vi "Periodic Tasks.vi"(8 "error in":errorcluster) -> ()   [LabVIEW 2018]
doc: "This VI runs in parallel to other robot code. It can contain as many user-defined periodic loops as you need. These can carry out PID or other sorts of timed response."
uses:
  <vilib>/Rock Robotics/WPI/Utilities/WPI_GetSetVariantRefNum.vi
  Robot Global Data.vi
panel:
  out "Cargo Stop Current":dbl=10.0 format="%#_13g"
  out "Stop the grabber":bool
  out "Solenoid Voltage":dbl
  out "Input Voltage":dbl
  out "Compressor current (A)":dbl
  out "all currents (A)":dbl[](array[numeric]) caption="0\n1\n2\n3\n4\n5\n6\n7\n8\n9\n10\n11\n12\n13\n14\n15"
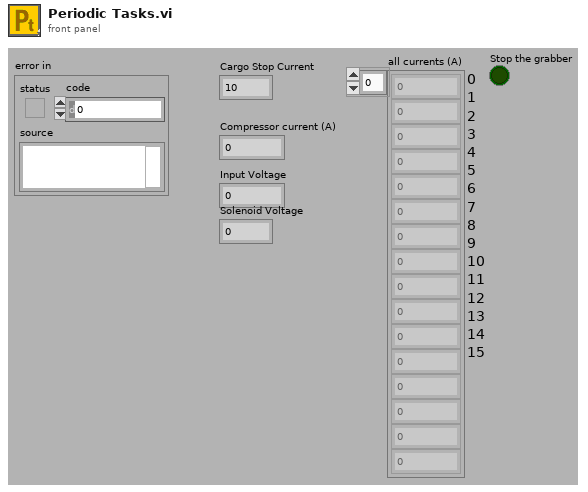
[diagram p1: front panel]
types:
  T1 = typedef "WPI_JoystickDevRef.ctl" = cluster{"Device":T2}
  T2 = typedef "WPI_JoystickDeviceEnum.ctl" = enum16{"USB 0", "USB 1", "USB 2", "USB 3", "USB 4", "USB 5"}
  T3 = cluster{"JoystickDevRef":T1, "JoystickDevRef":T1}
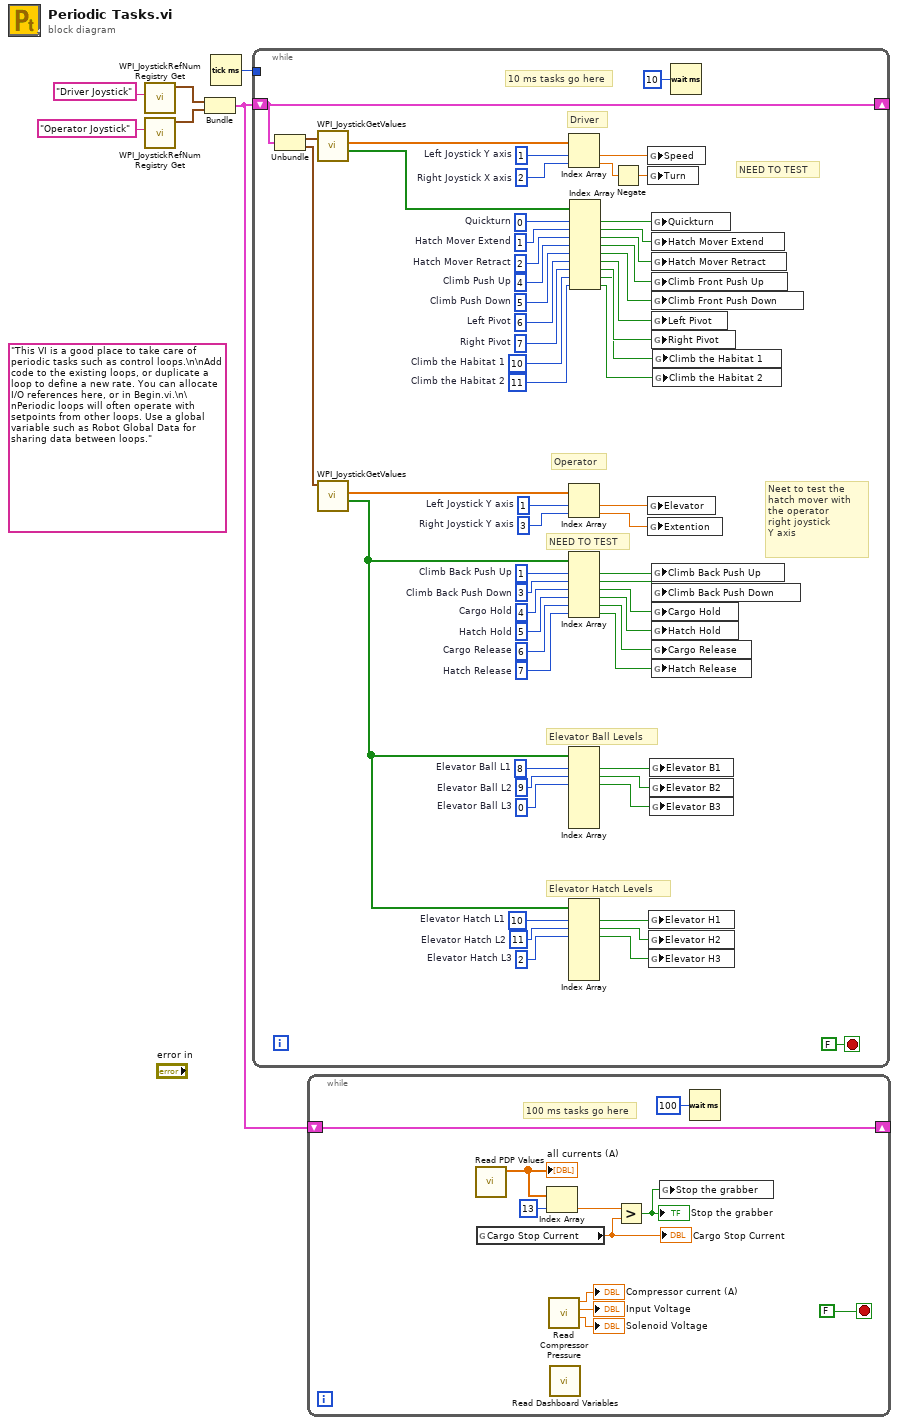
[diagram p0: block diagram]
diagram:
  (unwired) "This VI is a good place to take care of periodic tasks such as control loops.\n\nAdd code to the existing loops, or duplicate a loop to define a new rate. You can allocate I/O references here, or in Begin.vi.\n\nPeriodic loops will often operate with setpoints from other loops. Use a global variable such as Robot Global Data for sharing data between loops."
  n1 = call <vilib>:"WPI_JoystickRefNum Registry Get.vi"("refnum name"="Driver Joystick") -> ("JoystickDevRef"=w3:T1)  [unwired: 1 in, 9 out]
  n2 = call <vilib>:"WPI_JoystickRefNum Registry Get.vi"("refnum name"="Operator Joystick") -> ("JoystickDevRef"=w1:T1)  [unwired: 1 in, 9 out]
  n3 = Bundle("JoystickDevRef"=w3, "JoystickDevRef"=w1) -> (w2:T3)  [unwired: 1 in]
  n4 = Tick Count (ms)() -> (millisecond timer value=w5:u32)
  n5 = while {
    shift-right: [w61] -> _
    shift-left: w2 -> [w61]
    tunnel: w5 -> [_]
    stop <- FALSE stop-if-true
    w7 = 11  # Climb the Habitat 2
    w10 = 10  # Climb the Habitat 1
    w15 = 2  # Elevator Hatch L3
    w16 = 11  # Elevator Hatch L2
    w17 = 10  # Elevator Hatch L1
    w20 = 0  # Elevator Ball L3
    w19 = 9  # Elevator Ball L2
    w18 = 8  # Elevator Ball L1
    w25 = 3  # Right Joystick Y axis
    w29 = 7  # Right Pivot
    w28 = 6  # Left Pivot
    w35 = 5  # Climb Push Down
    w36 = 4  # Climb Push Up
    w43 = 7  # Hatch Release
    w44 = 6  # Cargo Release
    w45 = 5  # Hatch Hold
    w46 = 4  # Cargo Hold
    w47 = 3  # Climb Back Push Down
    w48 = 1  # Climb Back Push Up
    w50 = 1  # Left Joystick Y axis
    w51 = 2  # Hatch Mover Retract
    w52 = 1  # Hatch Mover Extend
    w53 = 0  # Quickturn
    w56 = 2  # Right Joystick X axis
    w57 = 1  # Left Joystick Y axis
    # "Elevator Hatch Levels"
    # "Elevator Ball Levels"
    # "10 ms tasks go here"
    # "Neet to test the\nhatch mover with\nthe operator \nright joystick\nY axis"
    # "Operator"
    # "Driver"
    # "NEED TO TEST"
    # "NEED TO TEST"
    n6 = Unbundle(w61) -> ("JoystickDevRef"=w60:T1, "JoystickDevRef"=w58:T1)
    n7 = call <vilib>:"WPI_JoystickGetValues.vi"("JoystickDevRef"=w60) -> ("Buttons"=w62:bool[], "Axes"=w64:dbl[])  [unwired: 6 in, 3 out]
    n8 = call <vilib>:"WPI_JoystickGetValues.vi"("JoystickDevRef"=w58) -> ("Buttons"=w11:bool[], "Axes"=w59:dbl[])  [unwired: 6 in, 3 out]
    n9 = Index Array(array=w64, index #1=w57, index #2=w56) -> (element #1=w55:dbl, element #2=w54:dbl)
    n10 = Index Array(array=w59, index #1=w50, index #2=w25) -> (element #1=w49:dbl, element #2=w24:dbl)
    n11 = Index Array(array=w11, index #1=w48, index #2=w47, index #3=w46, index #4=w45, index #5=w44, index #6=w43) -> (element #1=w42:bool, element #2=w41:bool, element #3=w40:bool, element #4=w39:bool, element #5=w38:bool, element #6=w37:bool)
    n12 = Index Array(array=w11, index #1=w18, index #2=w19, index #3=w20) -> (element #1=w21:bool, element #2=w22:bool, element #3=w23:bool)  [unwired: 5 in, 5 out]
    n13 = Index Array(array=w11, index #1=w17, index #2=w16, index #3=w15) -> (element #1=w14:bool, element #2=w13:bool, element #3=w12:bool)  [unwired: 5 in, 5 out]
    n14 = Index Array(array=w62, index #1=w53, index #2=w52, index #3=w51, index #4=w36, index #5=w35, index #6=w28, index #7=w29, index #8=w10, index #9=w7) -> (element #1=w34:bool, element #2=w33:bool, element #3=w32:bool, element #4=w31:bool, element #5=w30:bool, element #6=w26:bool, element #7=w27:bool, element #8=w9:bool, element #9=w8:bool)
    n15 = Negate(x=w54) -> (-x=w63:dbl)
    n16 = global write "Robot Global Data.vi" "Speed"(w55) -> ()
    n17 = global write "Robot Global Data.vi" "Turn"(w63) -> ()
    n18 = global write "Robot Global Data.vi" "Elevator"(w49) -> ()
    n19 = global write "Robot Global Data.vi" "Extention"(w24) -> ()
    n20 = global write "Robot Global Data.vi" "Elevator H1"(w14) -> ()
    n21 = global write "Robot Global Data.vi" "Elevator H2"(w13) -> ()
    n22 = global write "Robot Global Data.vi" "Elevator H3"(w12) -> ()
    n23 = global write "Robot Global Data.vi" "Elevator B1"(w21) -> ()
    n24 = global write "Robot Global Data.vi" "Elevator B2"(w22) -> ()
    n25 = global write "Robot Global Data.vi" "Elevator B3"(w23) -> ()
    n26 = global write "Robot Global Data.vi" "Quickturn"(w34) -> ()
    n27 = global write "Robot Global Data.vi" "Hatch Mover Extend"(w33) -> ()
    n28 = global write "Robot Global Data.vi" "Hatch Mover Retract"(w32) -> ()
    n29 = global write "Robot Global Data.vi" "Climb Front Push Up"(w31) -> ()
    n30 = global write "Robot Global Data.vi" "Climb Front Push Down"(w30) -> ()
    n31 = global write "Robot Global Data.vi" "Left Pivot"(w26) -> ()
    n32 = global write "Robot Global Data.vi" "Right Pivot"(w27) -> ()
    n33 = global write "Robot Global Data.vi" "Climb Back Push Up"(w42) -> ()
    n34 = global write "Robot Global Data.vi" "Climb Back Push Down"(w41) -> ()
    n35 = global write "Robot Global Data.vi" "Cargo Hold"(w40) -> ()
    n36 = global write "Robot Global Data.vi" "Hatch Hold"(w39) -> ()
    n37 = global write "Robot Global Data.vi" "Cargo Release"(w38) -> ()
    n38 = global write "Robot Global Data.vi" "Hatch Release"(w37) -> ()
    n39 = global write "Robot Global Data.vi" "Climb the Habitat 1"(w9) -> ()
    n40 = global write "Robot Global Data.vi" "Climb the Habitat 2"(w8) -> ()
    n41 = Wait (ms)(milliseconds to wait=u32 10) -> ()  [unwired: 1 out]
  }
  n42 = while {
    shift-right: [w75] -> _
    shift-left: w2 -> [w75]
    stop <- FALSE stop-if-true
    # "100 ms tasks go here"
    n43 = call "Read PDP Values.vi"() -> ("all currents (A)"=w69:dbl[])  [unwired: 11 in]
    "all currents (A)" <- w69
    n44 = global read "Robot Global Data.vi" "Cargo Stop Current"() -> (w71:dbl)
    "Cargo Stop Current" <- w71
    n45 = Index Array(array=w69, index=13) -> (element=w68:dbl)
    n46 = call "Read Compressor Pressure.vi"() -> ("Solenoid Voltage"=→"Solenoid Voltage":dbl, "Input Voltage"=→"Input Voltage":dbl, "Compressor current (A)"=→"Compressor current (A)":dbl)  [unwired: 9 in]
    n47 = call "Read Dashboard Variables.vi"() -> ()  [unwired: 12 in]
    n48 = Greater?(x=w68, y=w71) -> (0:w70:bool)
    "Stop the grabber" <- w70
    n49 = global write "Robot Global Data.vi" "Stop the grabber"(w70) -> ()
    n50 = Wait (ms)(milliseconds to wait=u32 100) -> ()  [unwired: 1 out]
  }
